vi "Slave.vi"() -> ()   [LabVIEW 2018]
panel:
  out "时间戳":u64 format="%016x"
  out "帧号":u16 format="%04x"
  in  "从站IP":string="192.168.3.100"
  in  "停止":bool
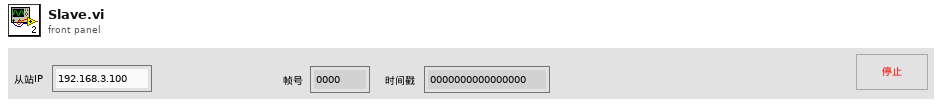
[diagram p1: front panel]
types:
  T1 = cluster{"主站IP":u32, "组号":u8, "帧号":u16, "时间戳":u64}
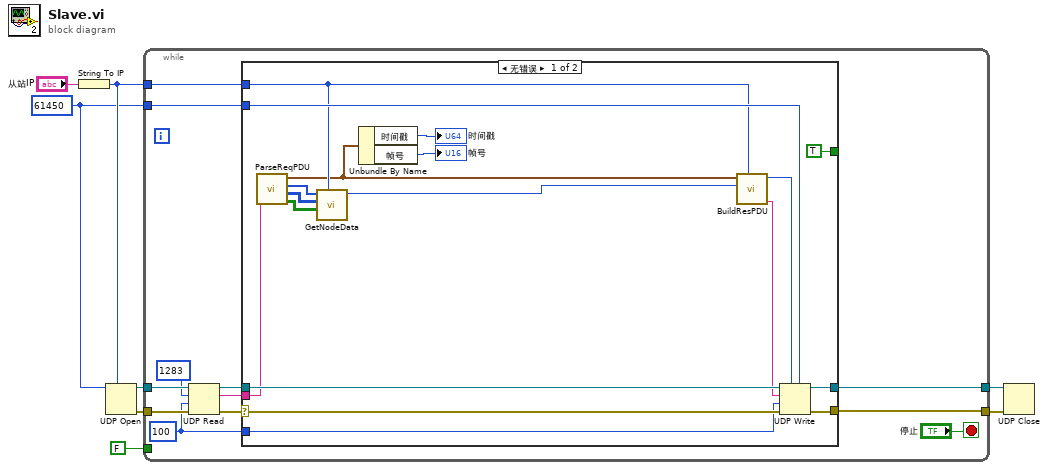
[diagram p0: block diagram]
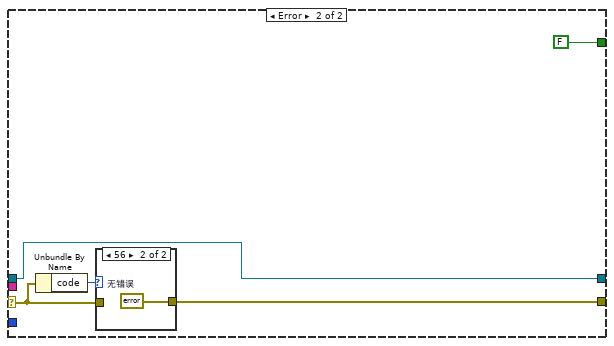
[diagram p2: hidden frame]
diagram:
  w2 = u16 61450 ("端口")
  n1 = String To IP(1:"从站IP") -> (0:w3:u32)
  n2 = UDP Open(7:w3, 11:w2) -> (port=w8:refnum<k16>, 0:w6:errorcluster)  [unwired: 3 in, 1 out]
  n3 = while {
    tunnel: w8 -> [w20]
    tunnel: [w11] -> w7
    tunnel: w6 -> [w19]
    tunnel: [w16] -> w5
    tunnel: w3 -> [w13]
    tunnel: w2 -> [w12]
    tunnel: FALSE -> [_]
    stop <- "停止" stop-if-true
    w10 = 100 ("超时毫秒(25000)")
    n4 = UDP Read(connection ID=w20, max size (548)=1283 ("最大值(548)"), timeout ms (25000)=w10, 8:w19) -> (data out=w17:string, error out=w18:errorcluster, 3:w14:refnum<k16>)  [unwired: 2 out]
    n5 = case shown="无错误" w18 {
      selector: w18 -> [w37 w42]
      tunnel: w17 -> [w32 _]
      tunnel: [w36 w41] -> w16
      tunnel: [TRUE FALSE] -> _
      tunnel: w14 -> [w35 w39]
      tunnel: w13 -> [w29 _]
      tunnel: w12 -> [w33 _]
      tunnel: [w34 w39] -> w11
      tunnel: w10 -> [w24 _]
      frame No Error {
        n6 = call "ParseReqPDU.vi"("数据in"=w32) -> ("All RY"=w25:bool[][], "All RWw"=w26:u16[][], "从站IP组"=w28:u32[], "主站信息"=w23:T1)  [unwired: 7 in]
        n7 = call "GetNodeData.vi"("指定从站IP"=w29, "All RY in"=w25, "All RWw in"=w26, "从站IP组"=w28) -> ("占用站数"=w27:i32)  [unwired: 5 in, 2 out]
        n8 = Unbundle By Name(w23) -> ("时间戳"=→"时间戳":u64, "帧号"=→"帧号":u16)
        n9 = call "BuildResPDU.vi"("从站IP"=w29, "占用站数"=w27, "主站信息"=w23) -> ("输出字符串"=w31:string, "主站IP"=w30:u32)  [unwired: 7 in]
        n10 = UDP Write(address=w30, port or service name=w33, connection ID=w35, data in=w31, 8:w37, 9:w24) -> (error out=w36:errorcluster, 3:w34:refnum<k16>)
      }
      frame Error {
        n11 = Unbundle By Name(w42) -> ("code"=w43:i32)
        n12 = case shown="56" w43 {
          tunnel: [w44 w45] -> w41
          tunnel: w42 -> [w44 _]
          frame Default {
          }
          frame 56 {
            w45 = errorcluster {"status"=FALSE, "code"=0, "source"=""}  # 无错误
          }
        }
      }
    }
  }
  n13 = UDP Close(connection ID=w7, 8:w5) -> ()  [unwired: 2 out]
